vi "RPC Get Reset Reason.vi"(6 "timeout (s)":dbl=60.0 format="%#_13g", 8 "error in (no error)":errorcluster, 11 "BLE address in":string) -> (0 "error out":errorcluster, 2 "Reason":u32, 3 "BLE address out":string)   [LabVIEW 2017]
uses:
  <vilib>/addons/InsightCM/Utilities/BleBackdoor/RPC Commands.ctl
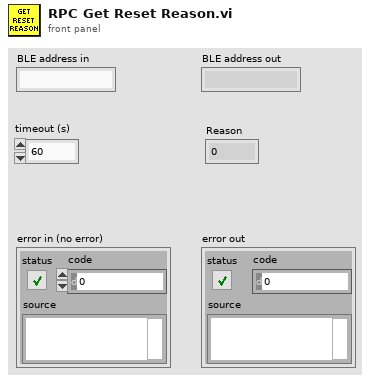
[diagram p1: front panel]
types:
  T1 = typedef "RPC Commands.ctl" = u16
  T2 = cluster{"response[0]":u8, "response[1]":u8, "response[2]":u8, "response[3]":u8}
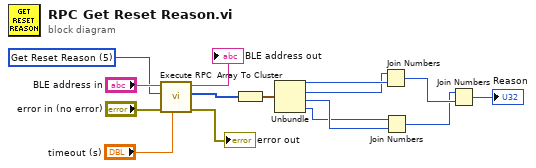
[diagram p0: block diagram]
diagram:
  w11 = T1 5 items=["Debug Print", "Configure ATECC", "Set Signed Identity", "Erase Bonds and Power Off", "Get Spider Cal Constants", "Get Reset Reason"] ("RPC Command")
  n1 = call <vilib>:"Execute RPC.vi"("timeout (s)"="timeout (s)", "error in (no error)"="error in (no error)", "RPC Command"=w11, "target endpoint MAC address in"="BLE address in") -> ("error out"=→"error out":errorcluster, "response"=w10:u8[], "target endpoint MAC address out"=→"BLE address out":string)  [unwired: 5 in]
  n2 = Array To Cluster(array=w10) -> (cluster=w9:T2)
  n3 = Unbundle(w9) -> ("response[0]"=w8:u8, "response[1]"=w7:u8, "response[2]"=w6:u8, "response[3]"=w5:u8)
  n4 = Join Numbers(hi=w7, lo=w8) -> ((hi.lo)=w4:u16)
  n5 = Join Numbers(hi=w5, lo=w6) -> ((hi.lo)=w3:u16)
  n6 = Join Numbers(hi=w3, lo=w4) -> ((hi.lo)=→"Reason":u32)
